vi "Variables Write for Tension Control.vi"(9 "RPM":dbl[](array[numeric]), 10 "Measured Tension":dbl[](array[numeric]), 11 "Cable Length in":dbl[](array[numeric])) -> ()   [LabVIEW 2021]
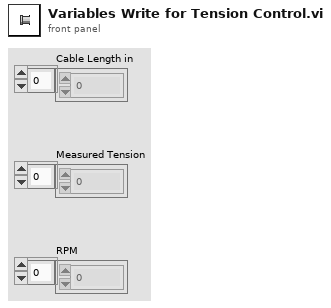
[diagram p1: front panel]
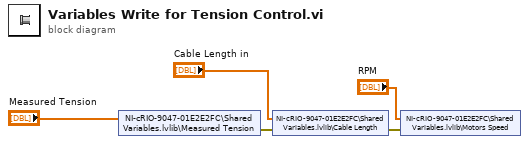
[diagram p0: block diagram]
diagram:
  n1 = shared-variable "NI-cRIO-9047-01E2E2FC\\Shared Variables.lvlib\\Measured Tension"("Measured Tension") -> (error out=w2:errorcluster)  [unwired: 1 in]
  n2 = shared-variable "NI-cRIO-9047-01E2E2FC\\Shared Variables.lvlib\\Cable Length"("Cable Length in", error in=w2) -> (error out=w1:errorcluster)
  n3 = shared-variable "NI-cRIO-9047-01E2E2FC\\Shared Variables.lvlib\\Motors Speed"("RPM", error in=w1) -> ()  [unwired: 1 out]
